vi "Save.vi"(8 "error in (no error)":errorcluster, 10 "Elements changed":string[](array[string]), 11 "ConfigManager.Text in":refnum<class "ConfigManager.Text.lvclass">) -> (0 "error out":errorcluster, 1 "success":bool, 3 "ConfigManager.Text out":refnum<class "ConfigManager.Text.lvclass">)   [LabVIEW 2013, in "CfgManager.Text.lvlib" / "ConfigManager.Text.lvclass"]
uses:
  ConfigManager.Text.lvclass
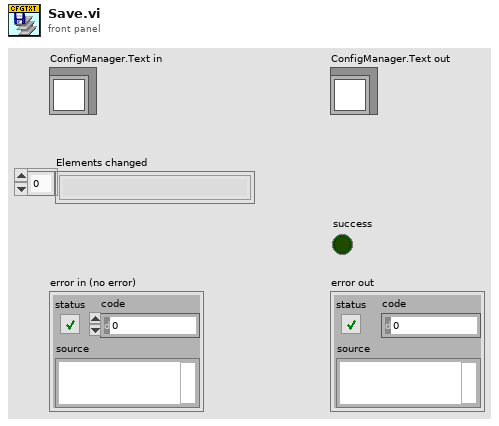
[diagram p1: front panel]
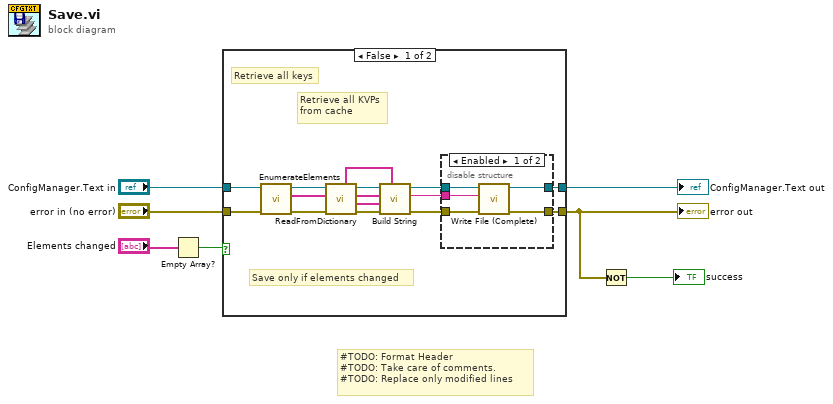
[diagram p0: block diagram]
diagram:
  # "#TODO: Format Header\n#TODO: Take care of comments.\n#TODO: Replace only modified lines"
  n1 = Empty Array?(array="Elements changed") -> (empty?=w1:bool)
  n2 = case shown="False" w1 {
    tunnel: "error in (no error)" -> [w12 w30]
    tunnel: "ConfigManager.Text in" -> [w10 w31]
    tunnel: [w9 w31] -> w5
    tunnel: [w8 w30] -> w4
    frame False {
      # "Save only if elements changed"
      # "Retrieve all KVPs\nfrom cache"
      # "Retrieve all keys"
      n3 = call-dynamic "EnumerateElements.vi"("error in (no error)"=w12, "ConfigManager.Text in"=w10) -> ("error out"=w14:errorcluster, "keys"=w22:string[], "ConfigManager.Text out"=w13:refnum<class "ConfigManager.Text.lvclass">)  [unwired: 7 in]
      n4 = call "ReadFromDictionary.vi"("error in (no error)"=w14, "Keys"=w22, "ConfigManager.Text in"=w13) -> ("error out"=w16:errorcluster, "Values"=w21:string[], "Keys out"=w20:string[], "ConfigManager.Text out"=w15:refnum<class "ConfigManager.Text.lvclass">, "Section"=w11:string[])  [unwired: 3 in, 1 out]
      n5 = call-dynamic "Build String.vi"("Section"=w11, "error in (no error)"=w16, "Values"=w21, "Keys"=w20, "ConfigManager.Text in"=w15) -> ("error out"=w17:errorcluster, "Input String"=w19:string, "ConfigManager.Text out"=w18:refnum<class "ConfigManager.Text.lvclass">)  [unwired: 4 in]
      n6 = disable-structure shown="Enabled" {
        disable-tunnel: [w27 w29] -> w9
        disable-tunnel: [w26 w28] -> w8
        disable-tunnel: w17 -> [w25 w28]
        disable-tunnel: w18 -> [w24 w29]
        disable-tunnel: w19 -> [w23 _]
        frame Enabled {
          n7 = call "Write File (Complete).vi"("error in (no error)"=w25, "String"=w23, "ConfigManager.Text in"=w24) -> ("error out"=w26:errorcluster, "ConfigManager.Text out"=w27:refnum<class "ConfigManager.Text.lvclass">)  [unwired: 7 in]
        }
        frame Disabled {
        }
      }
    }
    frame True {
    }
  }
  "ConfigManager.Text out" <- w5
  "error out" <- w4
  n8 = Not(x=w4) -> (.not. x?=→"success":bool)
